vi "PDCGetAndDisplay.vi"(8 "error in (no error)":errorcluster, 9 "ChildNo":u32, 10 "DeviceNo":u32, 11 "DataDisplayQueue":refnum<queue>) -> (0 "error out":errorcluster, 3 "PDCAllStates":T1)   [LabVIEW 2015]
uses:
  TypeDefs/MessageCluster.ctl
  TypeDefs/PDCAllStates.ctl
  TypeDefs/PDCDisplay.ctl
  TypeDefs/PDCRecordStatus.ctl
  TypeDefs/PDCLists.ctl
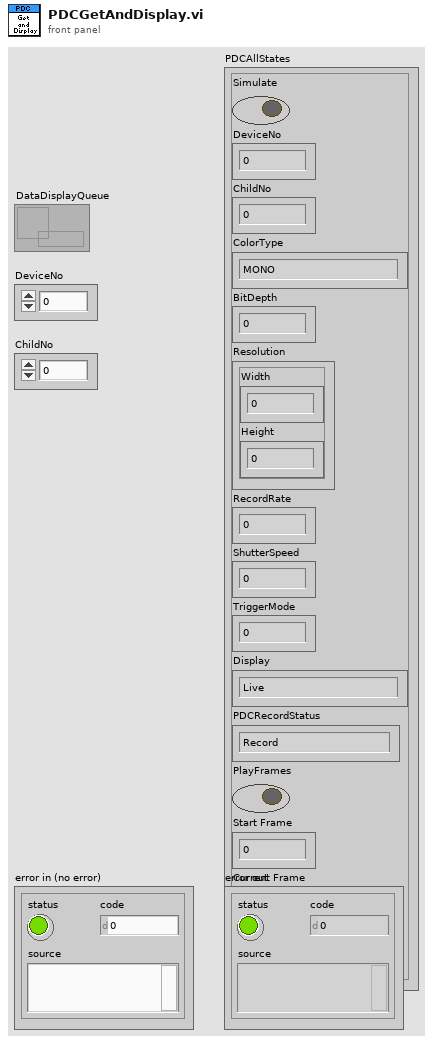
[diagram p1: front panel]
types:
  T1 = typedef "PDCAllStates.ctl" = cluster{"Simulate":bool, "DeviceNo":u32, "ChildNo":u32, "ColorType":enum16{"MONO", "COLOR"}, "BitDepth":i8, "Resolution":cluster{"Width":u32, "Height":u32}, "RecordRate":u32, "ShutterSpeed":u32, "TriggerMode":u32, "Display":T2, "PDCRecordStatus":T3, "PlayFrames":bool, "Start Frame":i32, "Current Frame":i32, "End Frame":i32}
  T2 = typedef "PDCDisplay.ctl" = enum16{"Live", "Memory", "LiveStop"}
  T3 = typedef "PDCRecordStatus.ctl" = enum16{"Record", "WaitingTRG", "Endless", "Recording"}
  T4 = typedef "PDCLists.ctl" = cluster{"ResolutionList":string[], "RecordRateList":string[], "ShutterSpeedList":string[], "TriggerModeList":string[]}
  T5 = typedef "PDCSetup.ctl" = cluster{"Color Type":enum16{"MONO", "COLOR"}, "Bit Depth":i8, "Resolution":u16, "Record Rate":u16, "Shutter Speed":u16, "Trigger Mode":u16, "Display":T2}
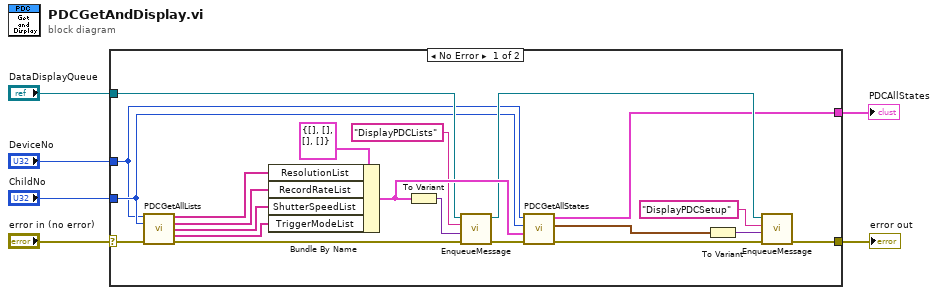
[diagram p0: block diagram]
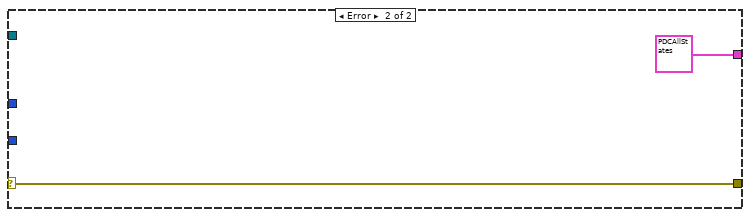
[diagram p2: hidden frame]
diagram:
  n1 = case shown="No Error" "error in (no error)" {
    selector: "error in (no error)" -> [w7 w29]
    tunnel: "DataDisplayQueue" -> [w17 _]
    tunnel: "ChildNo" -> [w15 _]
    tunnel: "DeviceNo" -> [w14 _]
    tunnel: [w13 T1 {"Simulate"=FALSE, "DeviceNo"=0, "ChildNo"=1, "ColorType"=enum."MONO", "BitDepth"=0, "Resolution"={"Width"=0, "Height"=0}, "RecordRate"=0, "ShutterSpeed"=0, "TriggerMode"=0, "Display"=enum."LiveStop", "PDCRecordStatus"=enum."Record", "PlayFrames"=FALSE, "Start Frame"=0, "Current Frame"=0, "End Frame"=0} ("PDCAllStates")] -> w3
    tunnel: [w8 w29] -> w2
    frame No Error {
      n2 = call "PDCGetAllLists.vi"("DeviceNo"=w14, "ChildNo"=w15, "error in (no error)"=w7) -> ("ResolutionList"=w23:string[], "RecordRateList"=w24:string[], "ShutterSpeedList"=w25:string[], "TriggerModeList"=w26:string[], "error out"=w22:errorcluster)  [unwired: 8 in]
      n3 = Bundle By Name(cluster=T4 {"ResolutionList"=[], "RecordRateList"=[], "ShutterSpeedList"=[], "TriggerModeList"=[]} ("PDCLists"), "ResolutionList"=w23, "RecordRateList"=w24, "ShutterSpeedList"=w25, "TriggerModeList"=w26) -> (w27:T4)
      n4 = To Variant(anything=w27) -> (Variant=w21:variant)
      n5 = call "EnqueueMessage.vi"("error in (no error)"=w22, "MessageData"=w21, "Message"="DisplayPDCLists", "MessageQueue"=w17) -> ("error out"=w16:errorcluster, "dupMessageQueue"=w18:refnum<queue>)  [unwired: 6 in]
      n6 = call "PDCGetAllStates.vi"("error in (no error)"=w16, "PDCLists"=w27, "ChildNo"=w15, "DeviceNo"=w14) -> ("error out"=w9:errorcluster, "PDC Setup"=w12:T5, "PDCAllStates"=w13:T1)  [unwired: 5 in]
      n7 = To Variant(anything=w12) -> (Variant=w10:variant)
      n8 = call "EnqueueMessage.vi"("error in (no error)"=w9, "MessageData"=w10, "Message"="DisplayPDCSetup", "MessageQueue"=w18) -> ("error out"=w8:errorcluster)  [unwired: 6 in, 1 out]
    }
    frame Error {
    }
  }
  "PDCAllStates" <- w3
  "error out" <- w2
